vi "Position Get.vi"(8 "error in (no error)":errorcluster) -> (0 "error out":errorcluster, 2 "Position":T1 {"z (mm)" format="%.1f"; "y (mm)" format="%.1f"; "x (mm)" format="%.1f"})   [LabVIEW 2021, in "Haptic Prog Interface.lvlib"]
doc: "Returns the position of the haptic pen in mm, and isn't dependent on the frame size.\n\n<b>Position:</b> Returns a cluster of the x, y, and z positions of the pen (in units of mm)."
uses:
  Users/cjwel/Documents/GitHub/Haptic-Programming-Interface/LabVIEW VIs/Haptic Prog Interface/Haptic Prog Interface.lvlib
  Haptic-Programming-Interface/src/x64/Debug/Haptic Programming Interface.dll
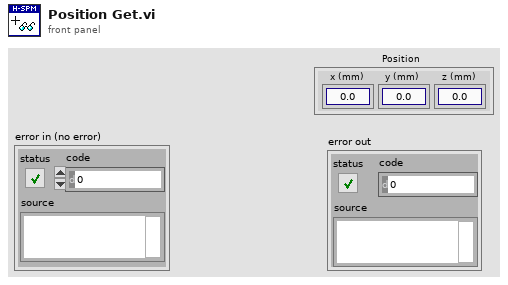
[diagram p1: front panel]
types:
  T1 = cluster{"x (mm)":dbl, "y (mm)":dbl, "z (mm)":dbl}
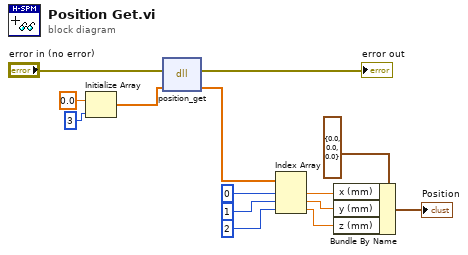
[diagram p0: block diagram]
diagram:
  n1 = Initialize Array(0.0 ("element"), 3 ("dimension size")) -> (w1:dbl[])
  n2 = dll-call lib="C:/Users/cjwel/Documents/GitHub/Haptic-Programming-Interface/src/x64/Debug/Haptic Programming Interface.dll" fn="position_get"(error in="error in (no error)", "output"=w1) -> (error out=→"error out":errorcluster, "output"=w12:dbl[])  [unwired: 3 in, 1 out]
  n3 = Index Array(array=w12, index #1=0 ("index"), index #2=1 ("index"), index #3=2 ("index")) -> (element #1=w7:dbl, element #2=w6:dbl, element #3=w5:dbl)
  n4 = Bundle By Name(cluster=T1 {"x (mm)"=0.0, "y (mm)"=0.0, "z (mm)"=0.0} ("Position"), "x (mm)"=w7, "y (mm)"=w6, "z (mm)"=w5) -> (→"Position":T1)
